vi "CB Continious to Discrete SSM.vi"(11 "Cont SSM":T1) -> (3 "Discrete SSM":T1)   [LabVIEW 2020]
uses:
  CB State Space.ctl
  <vilib>/Analysis/Matrix/Datatypes/RealMatrix.ctl
  <vilib>/Analysis/baseanly.llb/Real A x B.vi
  <vilib>/Analysis/baseanly.llb/Real Inverse Matrix.vi
  <vilib>/Analysis/Matrix/Numeric/Multiply/Multiply - RM,R.vi
  <vilib>/Analysis/Matrix/Numeric/Exponential/Exponential - RM.vi
  <vilib>/Analysis/7linalg.llb/Create Special Real Matrix.vi
  <vilib>/Analysis/Matrix/Numeric/Subtract/Subtract - RM,RM.vi
  <vilib>/Analysis/Matrix/NI_Matrix.lvlib
  <vilib>/Analysis/NI_AALPro.lvlib
  <vilib>/Analysis/NI_AALBase.lvlib
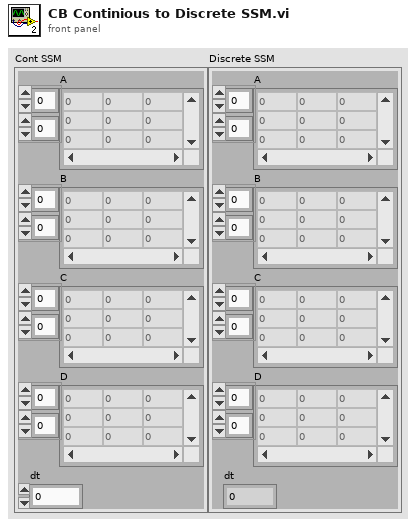
[diagram p1: front panel]
types:
  T1 = typedef "CB State Space.ctl" = cluster{"A":T2, "B":T2, "C":T2, "D":T2, "dt":dbl}
  T2 = typedef "NI_Matrix.lvlib/RealMatrix.ctl" = dbl[][]
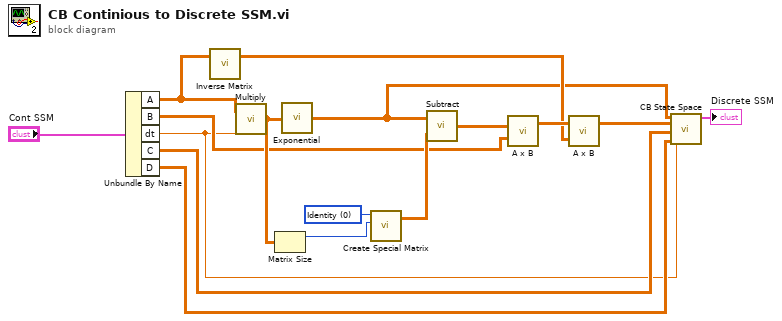
[diagram p0: block diagram]
diagram:
  w14 = 0 items=["Identity", "Diagonal", "Toeplitz", "Vandermonde", "Companion", "Hankel", "Hadamard", "Wilkinson", "Hilbert", "Inverse Hilbert", "Rosser", "Pascal"] ("matrix type")
  n1 = Unbundle By Name("Cont SSM") -> ("A"=w15:T2, "B"=w9:T2, "dt"=w2:dbl, "C"=w4:T2, "D"=w3:T2)
  n2 = call-poly <vilib>:"Inverse Matrix.vi"("Input Matrix"=w15) -> ("Inverse Matrix"=w7:T2)  [unwired: 1 in, 1 out]
  n3 = call-poly <vilib>:"Multiply.vi"("Real Scalar c"=w2, "Real Matrix A"=w15) -> ("A * c"=w13:T2)
  n4 = Matrix Size(0:w13) -> (1:w12:i32)  [unwired: 1 out]
  n5 = call-poly <vilib>:"Exponential.vi"("Real Matrix A"=w13) -> ("e^A"=w6:T2)
  n6 = call-poly <vilib>:"Create Special Matrix.vi"("matrix type"=w14, "matrix size"=w12) -> ("Special Matrix"=w11:T2)  [unwired: 3 in, 1 out]
  n7 = call-poly <vilib>:"Subtract.vi"("Real Matrix B"=w11, "Real Matrix A"=w6) -> ("A - B"=w10:T2)
  n8 = call-poly <vilib>:"A x B.vi"("B"=w9, "A"=w10) -> ("A x B"=w8:T2)  [unwired: 1 out]
  n9 = call-poly <vilib>:"A x B.vi"("B"=w7, "A"=w8) -> ("A x B"=w5:T2)  [unwired: 1 out]
  n10 = call "CB State Space.vi"("dt"=w2, "D"=w3, "C"=w4, "B"=w5, "A"=w6) -> ("State Space Model"=→"Discrete SSM":T1)  [unwired: 5 in, 1 out]
